vi "Remove Element.vi"(8 "error in (no error)":errorcluster, 10 "Index":i32=-1, 11 "ControlArray in":refnum<class "ControlArray.lvclass">) -> (0 "error out":errorcluster, 2 "Removed Value":variant, 3 "ControlArray out":refnum<class "ControlArray.lvclass">)   [LabVIEW 2020, in "Control Array.lvlib" / "ControlArray.lvclass"]
uses:
  ControlArray.lvclass
  ControlArray.lvclass/ControlArray.ctl
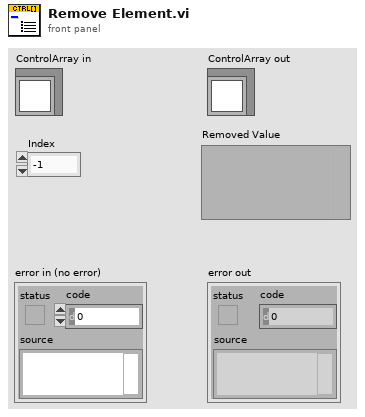
[diagram p1: front panel]
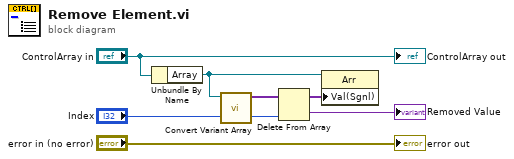
[diagram p0: block diagram]
diagram:
  n1 = Unbundle By Name("ControlArray in") -> ("Array"=w3:refnum<vi>)
  n2 = call "Convert Variant Array.vi"("Array"=w3) -> ("Variant Array"=w4:variant[])  [unwired: 9 in, 1 out]
  n3 = Delete From Array(array=w4, index="Index") -> (deleted portion=→"Removed Value":variant, array with subset deleted=w5:variant[])  [unwired: 1 in]
  n4 = property class="Arr"(reference=w3, "Val(Sgnl)"=w5) -> ()  [unwired: 1 in, 2 out]
  "error out" <- "error in (no error)"
  "ControlArray out" <- "ControlArray in"
